vi "Tolva de arena.vi"() -> ()   [LabVIEW 2012]
panel:
  out "400":bool
  out "200":bool
  out "100":bool
  out "50":bool
  in  "300":bool
  in  "250":bool
  in  "150":bool
  in  "50":bool
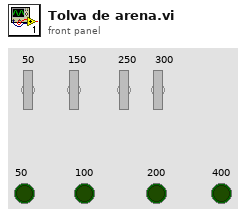
[diagram p1: front panel]
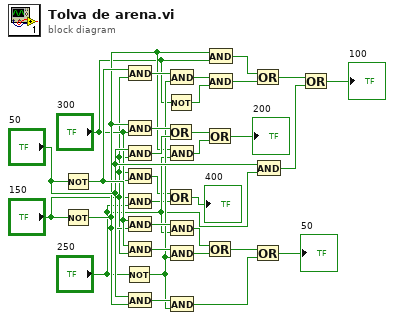
[diagram p0: block diagram]
diagram:
  n1 = Not(x="50") -> (.not. x?=w23:bool)
  n2 = Not(x="150") -> (.not. x?=w7:bool)
  n3 = Not(x="250") -> (.not. x?=w8:bool)
  n4 = And(x=w23, y="150") -> (x .and. y?=w21:bool)
  n5 = And(x=w7, y="300") -> (x .and. y?=w15:bool)
  n6 = And(x="50", y="150") -> (x .and. y?=w14:bool)
  n7 = And(x="150", y="300") -> (x .and. y?=w3:bool)
  n8 = And(x="150", y="250") -> (x .and. y?=w2:bool)
  n9 = And(x=w23, y=w7) -> (x .and. y?=w31:bool)
  n10 = And(x=w23, y="150") -> (x .and. y?=w30:bool)
  n11 = And(x="50", y=w7) -> (x .and. y?=w29:bool)
  n12 = Not(x="300") -> (.not. x?=w22:bool)
  n13 = Or(x=w15, y=w14) -> (x .or. y?=w13:bool)
  n14 = Or(x=w3, y=w2) -> (x .or. y?=→"400":bool)
  n15 = And(x=w21, y=w8) -> (x .and. y?=w10:bool)
  n16 = And(x=w7, y="250") -> (x .and. y?=w12:bool)
  n17 = And(x=w31, y="250") -> (x .and. y?=w28:bool)
  n18 = And(x=w30, y=w8) -> (x .and. y?=w27:bool)
  n19 = And(x=w29, y=w8) -> (x .and. y?=w25:bool)
  n20 = Or(x=w13, y=w12) -> (x .or. y?=→"200":bool)
  n21 = Or(x=w28, y=w27) -> (x .or. y?=w26:bool)
  n22 = And(x=w7, y="300") -> (x .and. y?=w20:bool)
  n23 = And(x=w10, y=w22) -> (x .and. y?=w19:bool)
  n24 = Or(x=w20, y=w19) -> (x .or. y?=w18:bool)
  n25 = Or(x=w26, y=w25) -> (x .or. y?=→"50":bool)
  n26 = And(x="50", y="250") -> (x .and. y?=w17:bool)
  n27 = Or(x=w18, y=w17) -> (x .or. y?=→"100":bool)
